vi "temp_FlpLib ResistorItoV.vi"(1 "R":sgl, 7 "Current":sgl) -> (8 "Voltage":sgl)   [LabVIEW 2016]
uses:
  <userlib>/_NI FLP Library/FPGA/outsideSCTL/FlpLib Multiply Shared Instance 0.vi
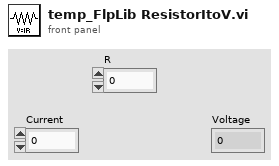
[diagram p1: front panel]
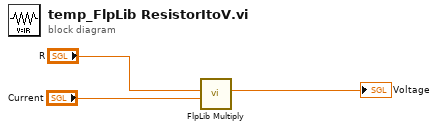
[diagram p0: block diagram]
diagram:
  n1 = call-poly <userlib>:"FlpLib Multiply.vi"("y"="Current", "x"="R") -> ("x*y"=→"Voltage":sgl)  [unwired: 5 in]
